vi "Remove Unused References.vi"(8 "error in (no error)":errorcluster, 10 "Channels.REF":T1 {"Roll-Off" min=1; "TC" min=0.0001 format="%#_3p"; "Phase" format="%#_3g"; "Frequency" min=0.0001 max=200000.0 format="%#_6p"; "Channel" min=1}, 11 "Channels.AI":T3 {"reference index" min=1; "References" items=["", "1", "2", "3", "4", "5", "6", "7", "8", "9"]; "Channel" min=1}) -> (0 "error out":errorcluster, 3 "Channels.AI out":T3 {"reference index" min=1; "References" items=["", "1", "2", "3", "4", "5", "6", "7", "8", "9"]; "Channel" min=1})   [LabVIEW 2020, in "Instrument.Lockin.lvlib" / "Instrument UI.Lockin.lvclass"]
uses:
  Instrument UI.Lockin.lvclass
  Instrument UI.Lockin.lvclass/Instrument UI.Lockin.ctl
  <userlib>/_OpenG.lib/array/array.llb/openg_array.lvlib
  <userlib>/_OpenG.lib/array/array.llb/Delete Elements from 1D Array (U16)__ogtk.vi
  Instrument.DAQ/Typedefs/AI.Channel--Cluster.ctl
  Instrument.DAQ/Instrument.DAQ.lvclass
  Instrument.DAQ/Typedefs/AI.Channel--Cluster--Array.ctl
  Instrument.DAQ/Typedefs/REF.Channel--Cluster.ctl
  Instrument.DAQ/Typedefs/REF.Channel--Cluster--Array.ctl
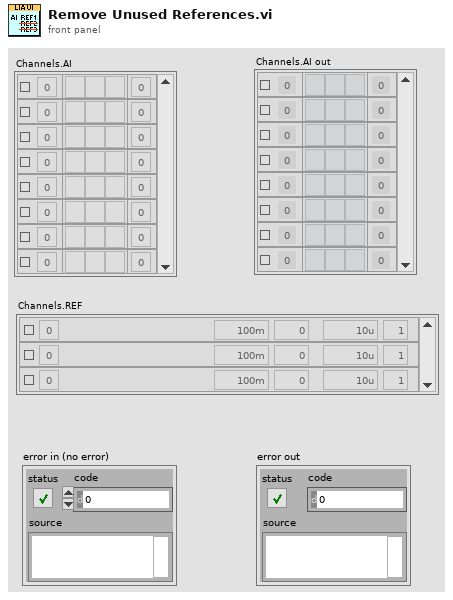
[diagram p1: front panel]
types:
  T1 = typedef "Instrument.Lockin.lvlib/Instrument.DAQ.lvclass/REF.Channel--Cluster--Array.ctl" = T2[]
  T2 = typedef "Instrument.Lockin.lvlib/Instrument.DAQ.lvclass/REF.Channel--Cluster.ctl" = cluster{"Enable?":bool, "Channel":i32, "Frequency":dbl, "Phase":dbl, "TC":dbl, "Roll-Off":i32}
  T3 = typedef "Instrument.Lockin.lvlib/Instrument.DAQ.lvclass/AI.Channel--Cluster--Array.ctl" = T4[]
  T4 = typedef "Instrument.Lockin.lvlib/Instrument.DAQ.lvclass/AI.Channel--Cluster.ctl" = cluster{"Enable?":bool, "Channel":i32, "References":u16[], "reference index":i32}
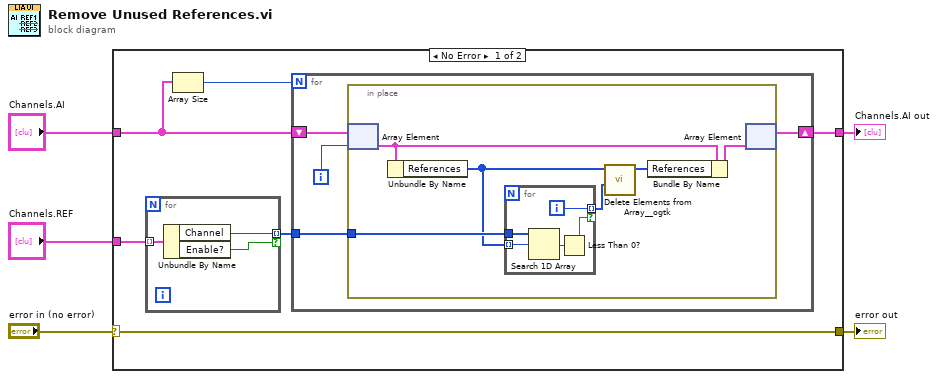
[diagram p0: block diagram]
diagram:
  n1 = case shown="No Error" "error in (no error)" {
    selector: "error in (no error)" -> [w6 w31]
    tunnel: [w7 w30] -> w5
    tunnel: [w6 w31] -> w3
    tunnel: "Channels.AI" -> [w8 w30]
    tunnel: "Channels.REF" -> [w10 _]
    frame No Error {
      n2 = for {
        tunnel: [w14] -> w11 mode=indexing if=w12
        tunnel: w10 -> [w13] mode=indexing
        n3 = Unbundle By Name(w13) -> ("Channel"=w14:i32, "Enable?"=w12:bool)
      }
      n4 = Array Size(array=w8) -> (size(s)=w9:i32)
      n5 = for {
        N: w9 -> [_]
        tunnel: w11 -> [w18]
        shift-right: [w16] -> w7
        shift-left: w8 -> [w17]
        i -> [w15]
        n6 = in-place {
          in-place-border: w18 -> [w24]
          n7 = in-place-array #1(w17, w15) -> (w20:T4)
          n8 = Unbundle By Name(w20) -> ("References"=w22:u16[])
          n9 = for {
            tunnel: w24 -> [w29]
            tunnel: w22 -> [w28] mode=indexing
            tunnel: [w26] -> w23 mode=indexing if=w25
            i -> [w26]
            n10 = Search 1D Array(1D array=w29, element=w28) -> (index of element=w27:i32)  [unwired: 1 in]
            n11 = Less Than 0?(x=w27) -> (x < 0?=w25:bool)
          }
          n12 = call-poly <userlib>:"Delete Elements from Array__ogtk.vi"("indices"=w23, "array"=w22) -> ("array w/ subset deleted"=w21:u16[])  [unwired: 8 in, 1 out]
          n13 = Bundle By Name(cluster=w20, "References"=w21) -> (w19:T4)
          n14 = in-place-array #1(w19) -> (w16:T3)  [unwired: 1 out]
        }
      }
    }
    frame Error {
    }
  }
  "error out" <- w3
  "Channels.AI out" <- w5
